vi "Language.vi"(3 "menu reference":refnum<k9>, 4 "LanguageFiles":T1) -> (1 "LanguageFiles Out":T1)   [LabVIEW 2020]
panel:
  in  "Cancel":bool
  in  "OK":bool
  in  "Ring":u16(ring) items=["Português (BR)", "English"]
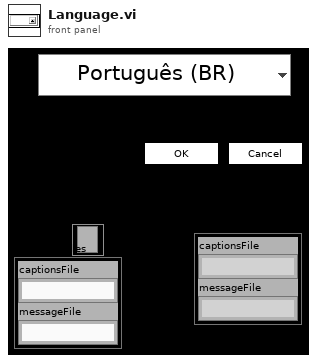
[diagram p1: front panel]
types:
  T1 = cluster{"captionsFile":string, "messageFile":string}
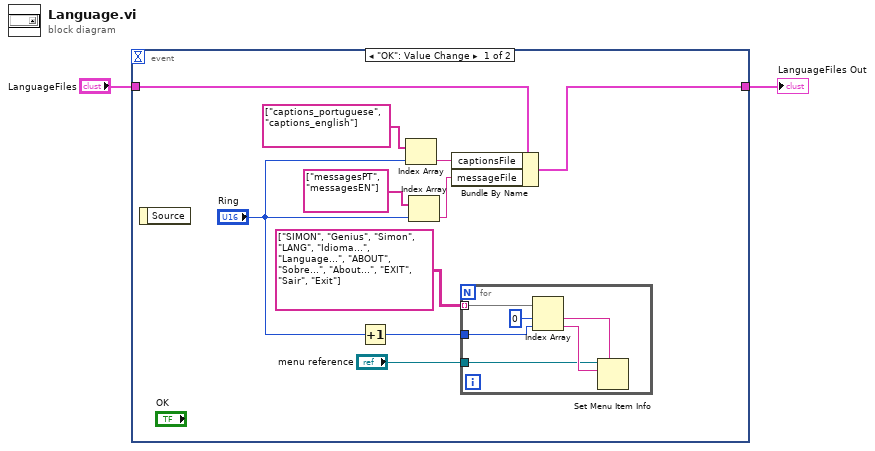
[diagram p0: block diagram]
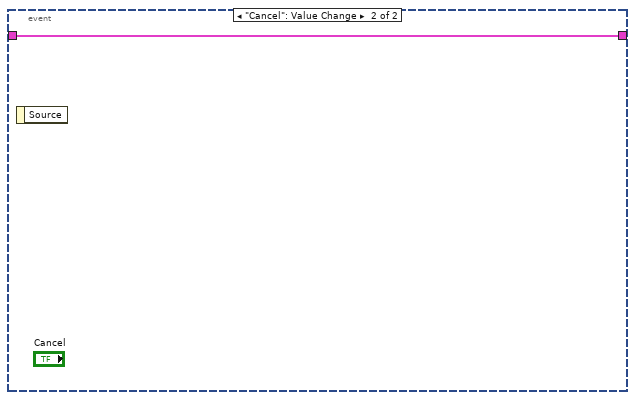
[diagram p2: hidden frame]
diagram:
  n1 = event shown="[0] \"OK\": Value Change" {
    selector: _ -> [_ _]
    dyn-events: _ -> [_ _]
    timeout: _ -> [_ _]
    tunnel: "LanguageFiles" -> [w4 w19]
    tunnel: [w3 w19] -> w1
    event "OK": Value Change {
      n2 = event-data() -> ()  [unwired: 1 in, 1 out]
      n3 = Increment(x="Ring") -> (x+1=w5:u16)
      n4 = Index Array(array=string[] ["captions_portuguese", "captions_english"] ("Captions File"), index="Ring") -> (element=w8:string)
      n5 = Index Array(array=string[] ["messagesPT", "messagesEN"] ("FileName (without extension)"), index="Ring") -> (element=w7:string)
      n6 = Bundle By Name(cluster=w4, "captionsFile"=w8, "messageFile"=w7) -> (w3:T1)
      n7 = for {
        tunnel: string[][] [["SIMON", "Genius", "Simon"], ["LANG", "Idioma...", "Language..."], ["ABOUT", "Sobre...", "About..."], ["EXIT", "Sair", "Exit"]] -> [w18] mode=indexing
        tunnel: w5 -> [w16]
        tunnel: "menu reference" -> [w13]
        n8 = Index Array(array=w18, index #1=0 ("index"), index #2=w16) -> (element #1=w17:string, element #2=w14:string)
        n9 = Set Menu Item Info(7:w17, 10:w14, 11:w13) -> ()  [unwired: 4 in, 2 out]
      }
    }
    event "Cancel": Value Change {
      n10 = event-data() -> ()  [unwired: 1 in, 1 out]
    }
  }
  "LanguageFiles Out" <- w1
